vi "Read Delivery Notifier.vi"(8 "error in (no error)":errorcluster, 11 "ReceiverState in":refnum<class "Connect Command.lvclass">) -> (0 "error out":errorcluster, 2 "Delivery Notifier":refnum<notifier>, 3 "ReceiverState out":refnum<class "Connect Command.lvclass">)   [LabVIEW 2013, in "Receiver.lvlib" / "Receive Commands Using State Actors.lvlib" / "Connect Command.lvlib" / "Connect Command.lvclass"]
uses:
  Connect Command/Connect Command.lvclass
  <vilib>/ActorFramework/Time-Delayed Send Message/Time-Delay Override Options.ctl
  Connect Command/Connect Command.lvclass/Connect Command.ctl
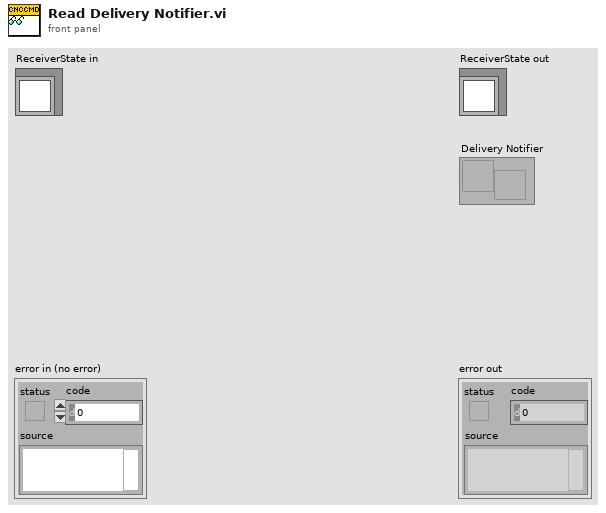
[diagram p1: front panel]
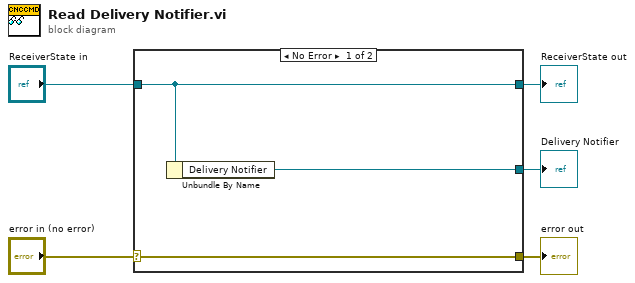
[diagram p0: block diagram]
diagram:
  n1 = case shown="No Error" "error in (no error)" {
    selector: "error in (no error)" -> [w8 w9]
    tunnel: [w8 w9] -> w4
    tunnel: [w7 w10] -> w2
    tunnel: "ReceiverState in" -> [w7 w10]
    tunnel: [w6 _] -> w1
    frame No Error {
      n2 = Unbundle By Name(w7) -> ("Delivery Notifier"=w6:refnum<notifier>)
    }
    frame Error {
    }
  }
  "error out" <- w4
  "ReceiverState out" <- w2
  "Delivery Notifier" <- w1
